vi "Temp2700GetCurrentPV.vi"(8 "error in":errorcluster, 10 "Current Temp":bool, 11 "VISA resource name":refnum<visa-resource-name>) -> (0 "error out":errorcluster, 2 "Temp":sgl, 5 "Data Valid":bool)   [LabVIEW 2016]
doc: "Read current presented value (Symbol: NPV)\nValue stored in D0001 register"
uses:
  <instrlib>/Samwontech TEMP2xxx/Samwontech TEMP2xxx.lvlib
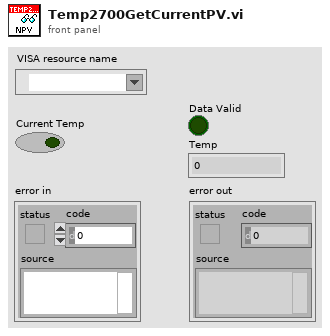
[diagram p1: front panel]
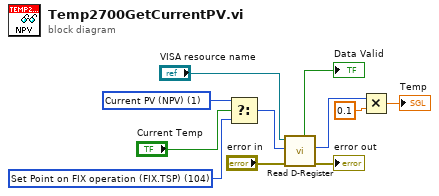
[diagram p0: block diagram]
diagram:
  w3 = u32 104 items=["Current PV (NPV)"=1, "Operation Control (COM.OPMODE)"=102, "Set Point on FIX operation (FIX.TSP)"=104, "Operation Mode (OP.MODE)"=106] ("D-Registers Map")
  w4 = u32 1 items=["Current PV (NPV)"=1, "Operation Control (COM.OPMODE)"=102, "Set Point on FIX operation (FIX.TSP)"=104, "Operation Mode (OP.MODE)"=106] ("D-Registers Map")
  n1 = Select(t=w4, s="Current Temp", f=w3) -> (s? t:f=w2:u32)
  n2 = call <instrlib>:"Read D-Register.vi"("error in"="error in", "D-register number"=w2, "VISA resource name"="VISA resource name") -> ("error out"=→"error out":errorcluster, "Data"=w7:i16, "Data Valid"=→"Data Valid":bool)  [unwired: 4 in, 2 out]
  n3 = Multiply(x=w7, y=0.1) -> (x*y=→"Temp":dbl)
